vi "Perform Lookup Table.vi"(0 "RFmx Instrument Handle In":refnum<k21> caption="Instrument Handle In", 1 "Selector String":string, 5 "SG Instrument Handle In":refnum<k15>, 7 "Waveform":T2={"Waveform Name"="Wfm", "Waveform"={"x0"=0.0, "dx"=0.0, "y"=[]}, "Signal Bandwidth (Hz)"=0.0, "PAPR (dB)"=0.0, "Burst Length (s)"=0.0, "Sample Rate"=0.0, "Burst Start Locations"=[], "Burst Stop Locations"=[], "Idle Duration Present?"=FALSE, "Runtime Scaling"=0.0, "Script"=""} {"Runtime Scaling" format="%#_6p"; "Sample Rate" format="%#_6p"; "Burst Length (s)" format="%#_6p"; "PAPR (dB)" format="%.2f"; "Signal Bandwidth (Hz)" format="%#_6p"; "Waveform"."y" format="%.2f"; "Waveform"."dx" format="%^.2e"; "Waveform"."x0" format="%^.2e"}, 11 "error in (no error)":errorcluster) -> (4 "RFmx Instrument Handle Out":refnum<k21> caption="Instrument Handle Out", 6 "SG Instrument Handle Out":refnum<k15>, 8 "Lookup Table Results":T1={"Post DPD Waveform"={"Waveform Name"="Wfm", "Waveform"={"x0"=0.0, "dx"=0.0, "y"=[]}, "Signal Bandwidth (Hz)"=0.0, "PAPR (dB)"=0.0, "Burst Length (s)"=0.0, "Sample Rate"=0.0, "Burst Start Locations"=[], "Burst Stop Locations"=[], "Idle Duration Present?"=FALSE, "Runtime Scaling"=0.0, "Script"=""}, "Input Powers (dBm)"=[], "Complex Gains (dB)"=[], "Power Offset (dB)"=-1.0} {"Post DPD Waveform"."Runtime Scaling" format="%#_6p"; "Post DPD Waveform"."Sample Rate" format="%#_6p"; "Post DPD Waveform"."Burst Length (s)" format="%#_6p"; "Post DPD Waveform"."PAPR (dB)" format="%.2f"; "Post DPD Waveform"."Signal Bandwidth (Hz)" format="%#_6p"; "Post DPD Waveform"."Waveform"."y" format="%.2f"; "Post DPD Waveform"."Waveform"."dx" format="%^.2e"; "Post DPD Waveform"."Waveform"."x0" format="%^.2e"; "Power Offset (dB)" format="%.2f"}, 15 "error out":errorcluster)   [LabVIEW 2016, in "RFmxDPD.lvlib"]
uses:
  RFmxDPD.lvlib
  SG/Typedefs/Waveform.ctl
  Typedefs/Lookup Table Results.ctl
  <vilib>/RFmx/SpecAn/mx/RFmxSpecAn.llb/RFmxSpecAn DPD Fetch Lookup Table.vi
  SG/SG.lvlib
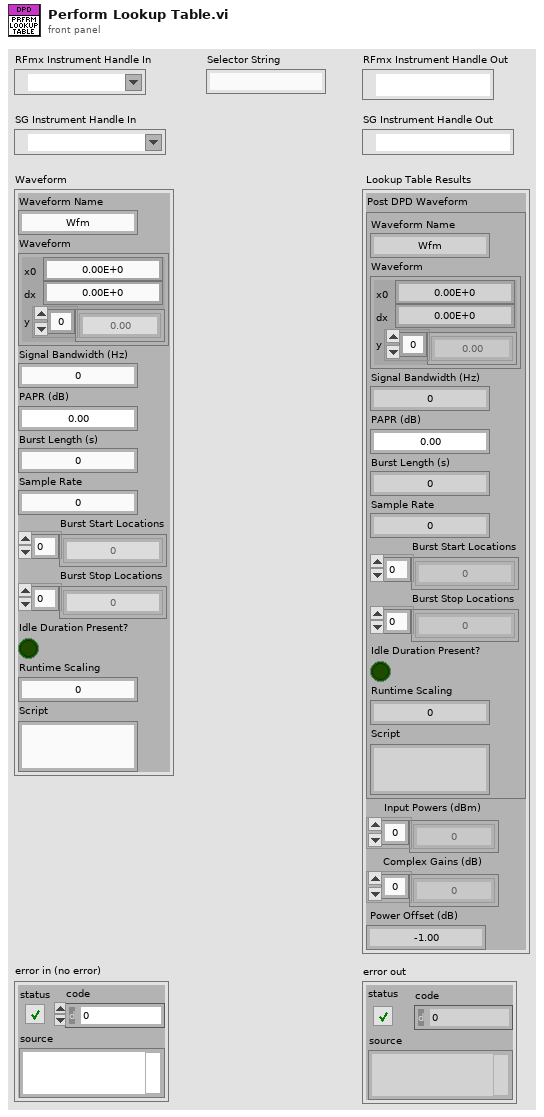
[diagram p1: front panel]
types:
  T1 = typedef "RFmxDPD.lvlib/Lookup Table Results.ctl" = cluster{"Post DPD Waveform":T2, "Input Powers (dBm)":sgl[], "Complex Gains (dB)":csg[], "Power Offset (dB)":dbl}
  T2 = typedef "SG.lvlib/Waveform.ctl" = cluster{"Waveform Name":string, "Waveform":cluster{"x0":dbl, "dx":dbl, "y":csg[]}, "Signal Bandwidth (Hz)":dbl, "PAPR (dB)":dbl, "Burst Length (s)":dbl, "Sample Rate":dbl, "Burst Start Locations":i32[], "Burst Stop Locations":i32[], "Idle Duration Present?":bool, "Runtime Scaling":dbl, "Script":string}
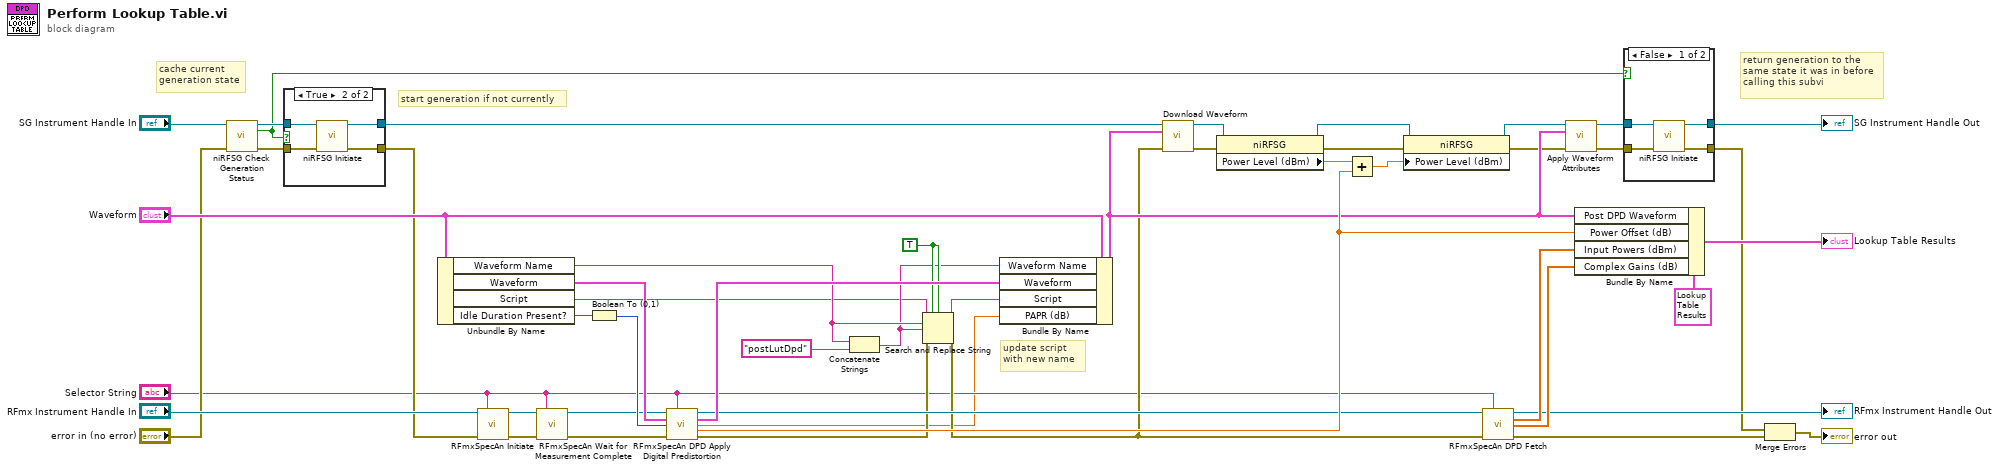
[diagram p0: block diagram]
diagram:
  w11 = TRUE ("replace all? (F)")
  # "cache current\ngeneration state"
  # "return generation to the\nsame state it was in before\ncalling this subvi"
  # "start generation if not currently"
  # "update script\nwith new name"
  n1 = call <instrlib>:"niRFSG Check Generation Status.vi"("instrument handle"="SG Instrument Handle In", "error in"="error in (no error)") -> ("instrument handle out"=w30:refnum<k15>, "done?"=w23:bool, "error out"=w31:errorcluster)  [unwired: 11 in]
  n2 = case shown="True" w23 {
    tunnel: w31 -> [w51 w54]
    tunnel: w30 -> [w50 w55]
    tunnel: [w50 w53] -> w29
    tunnel: [w51 w52] -> w28
    frame False {
    }
    frame True {
      n3 = call <instrlib>:"niRFSG Initiate.vi"("instrument handle"=w55, "error in"=w54) -> ("instrument handle out"=w53:refnum<k15>, "error out"=w52:errorcluster)  [unwired: 12 in]
    }
  }
  n4 = Unbundle By Name("Waveform") -> ("Waveform Name"=w10:string, "Waveform"=w48:cluster{"x0":dbl, "dx":dbl, "y":csg[]}, "Script"=w2:string, "Idle Duration Present?"=w3:bool)
  n5 = call <vilib>:"RFmxSpecAn Initiate.vi"("Instrument Handle In"="RFmx Instrument Handle In", "Selector String"="Selector String", "error in (no error)"=w28) -> ("Instrument Handle Out"=w6:refnum<k21>, "error out"=w27:errorcluster)  [unwired: 10 in, 1 out]
  n6 = call <vilib>:"RFmxSpecAn Wait for Measurement Complete.vi"("Instrument Handle In"=w6, "Selector String"="Selector String", "error in (no error)"=w27) -> ("Instrument Handle Out"=w5:refnum<k21>, "error out"=w7:errorcluster)  [unwired: 11 in]
  n7 = Boolean To (0,1)(Boolean=w3) -> (0, 1=w47:i16)
  n8 = call <vilib>:"RFmxSpecAn DPD Apply Digital Predistortion.vi"("Instrument Handle In"=w5, "Selector String"="Selector String", "Waveform In"=w48, "Idle Duration Present"=w47, "error in (no error)"=w7) -> ("Instrument Handle Out"=w21:refnum<k21>, "Waveform Out"=w34:cluster{"x0":dbl, "dx":dbl, "y":csg[]}, "PAPR (dB)"=w1:dbl, "Power Offset (dB)"=w38:dbl, "error out"=w13:errorcluster)  [unwired: 6 in]
  n9 = Concatenate Strings(w10, "postLutDpd" ("string")) -> (w9:string)
  n10 = Search and Replace String(replace all?=w11, case sensitive?=w11, input string=w2, search string=w10, replace string=w9, error in=w13) -> (result string=w8:string, error out=w12:errorcluster)  [unwired: 2 in, 2 out]
  n11 = Bundle By Name(cluster="Waveform", "Waveform Name"=w9, "Waveform"=w34, "Script"=w8, "PAPR (dB)"=w1) -> (w24:T2)
  n12 = call "Download Waveform.vi"("RFSG handle"=w29, "Waveform In"=w24, "error in (no error)"=w12) -> ("RFSG handle out"=w44:refnum<k15>, "error out"=w20:errorcluster)  [unwired: 11 in]
  n13 = property class="niRFSG"(reference=w44, error in=w20) -> (reference out=w45:refnum<k15>, error out=w19:errorcluster, "Power Level (dBm)"=w43:dbl)
  n14 = Add(x=w43, y=w38) -> (x+y=w42:dbl)
  n15 = property class="niRFSG"(reference=w45, error in=w19, "Power Level (dBm)"=w42) -> (reference out=w26:refnum<k15>, error out=w18:errorcluster)
  n16 = call-poly <vilib>:"RFmxSpecAn DPD Fetch.vi"("Instrument Handle In"=w21, "Selector String"="Selector String", "error in (no error)"=w12) -> ("Instrument Handle Out"=→"RFmx Instrument Handle Out":refnum<k21>, "Input Powers"=w40:sgl[], "Complex Gains"=w39:csg[], "error out"=w15:errorcluster)  [unwired: 9 in]
  n17 = call "Apply Waveform Attributes.vi"("RFSG Session In"=w26, "Waveform"=w24, "error in (no error)"=w18) -> ("RFSG Session Out"=w25:refnum<k15>, "error out"=w17:errorcluster)  [unwired: 11 in]
  n18 = Bundle By Name(cluster=T1 {"Post DPD Waveform"={"Waveform Name"="Wfm", "Waveform"={"x0"=0.0, "dx"=0.0, "y"=[]}, "Signal Bandwidth (Hz)"=0.0, "PAPR (dB)"=0.0, "Burst Length (s)"=0.0, "Sample Rate"=0.0, "Burst Start Locations"=[], "Burst Stop Locations"=[], "Idle Duration Present?"=FALSE, "Runtime Scaling"=0.0, "Script"=""}, "Input Powers (dBm)"=[], "Complex Gains (dB)"=[], "Power Offset (dB)"=-1.0} ("Lookup Table Results"), "Post DPD Waveform"=w24, "Power Offset (dB)"=w38, "Input Powers (dBm)"=w40, "Complex Gains (dB)"=w39) -> (→"Lookup Table Results":T1)
  n19 = case shown="False" w23 {
    tunnel: [w59 w61] -> w46
    tunnel: [w58 w60] -> w16
    tunnel: w25 -> [w57 w61]
    tunnel: w17 -> [w56 w60]
    frame False {
      n20 = call <instrlib>:"niRFSG Initiate.vi"("instrument handle"=w57, "error in"=w56) -> ("instrument handle out"=w59:refnum<k15>, "error out"=w58:errorcluster)  [unwired: 12 in]
    }
    frame True {
    }
  }
  "SG Instrument Handle Out" <- w46
  n21 = Merge Errors(w16, w15) -> (→"error out":errorcluster)
